vi "PH_Connection.VISA find Resources.vi"(5 "error in":errorcluster) -> (16 "VISA Information":T1(array[cluster]) {"Interface Information: Interface Type" items=["GPIB"=1, "VXI"=2, "GPIB-VXI"=3, "Serial"=4, "PXI"=5, "TCPIP"=6, "USB"=7, "FireWire"=9]}, 19 "error out":errorcluster)   [LabVIEW 2014, in "PH_Common.lvlib"]
doc: "This VI is forseen to select a string from an array of strings."
uses:
  PH_Common.lvlib
panel:
  in  "Find VISA Resources":bool
  in  "STOP":bool
  # "PCS"
  # "3.40"
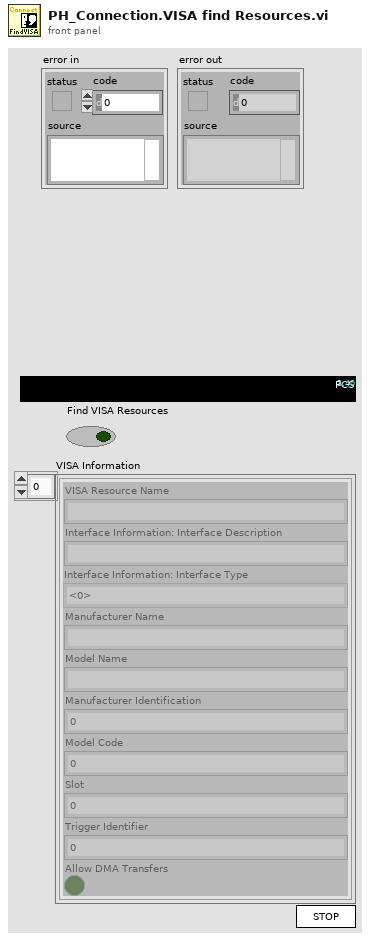
[diagram p1: front panel]
types:
  T1 = cluster{"VISA Resource Name":string, "Interface Information: Interface Description":string, "Interface Information: Interface Type":u16, "Manufacturer Name":string, "Model Name":string, "Manufacturer Identification":u16, "Model Code":u16, "Slot":i16, "Trigger Identifier":i16, "Allow DMA Transfers":bool}[]
  T2 = cluster{"VISA Resource Name":string, "Manufacturer Name":string, "Model Name":string, "Manufacturer Identification":u16, "Model Code":u16, "Slot":i16, "Trigger Identifier":i16, "Allow DMA Transfers":bool}[]
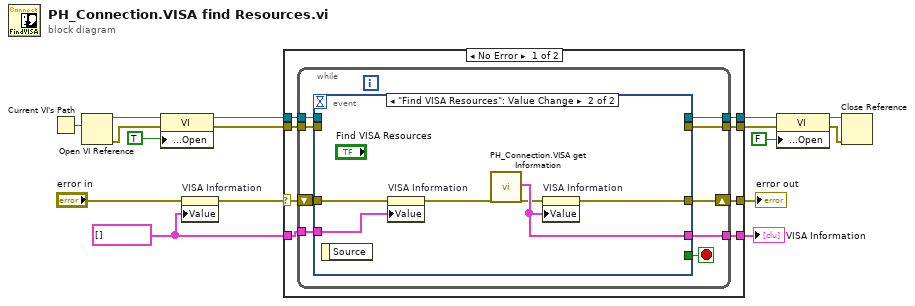
[diagram p0: block diagram]
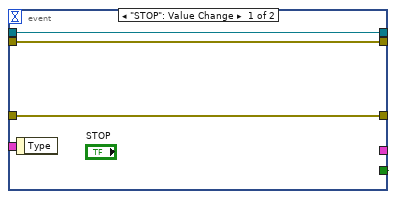
[diagram p2: hidden frame]
diagram:
  w1 = T1 [] ("VISA Information")
  n1 = Current VI's Path() -> (path=w15:path)
  n2 = Open VI Reference(vi path=w15) -> (vi reference=w14:refnum<vi>, error out=w8:errorcluster)  [unwired: 5 in]
  n3 = property class="VI"(reference=w14, error in=w8, "Front Panel Window:Open"=TRUE) -> (reference out=w12:refnum<vi>, error out=w6:errorcluster)
  n4 = property on="VISA Information" class="Arr (strict)"(error in="error in", "Value"=w1) -> (error out=w2:errorcluster)  [unwired: 1 in, 1 out]
  n5 = case shown="No Error" w2 {
    selector: w2 -> [w21 w47]
    tunnel: [w22 w47] -> w16
    tunnel: w12 -> [w24 w46]
    tunnel: [w23 w46] -> w10
    tunnel: w6 -> [w20 w45]
    tunnel: [w19 w45] -> w5
    tunnel: [w18 w44] -> w4
    tunnel: w1 -> [w17 w44]
    frame No Error {
      n6 = while {
        tunnel: w24 -> [w33]
        tunnel: [w32] -> w23
        shift-right: [w31] -> w22
        shift-left: w21 -> [w30]
        tunnel: w20 -> [w28]
        tunnel: [w27] -> w19
        tunnel: [w26] -> w18
        tunnel: w17 -> [w25]
        stop <- w29 stop-if-true
        n7 = event shown="[1] \"Find VISA Resources\": Value Change" {
          selector: _ -> [_ _]
          dyn-events: _ -> [_ _]
          timeout: _ -> [_ _]
          tunnel: [w37 _] -> w32
          tunnel: w33 -> [w37 _]
          tunnel: w30 -> [w36 w40]
          tunnel: [w36 w41] -> w31
          tunnel: [TRUE _] -> w29
          tunnel: w28 -> [w34 _]
          tunnel: [w34 _] -> w27
          tunnel: [_ w43] -> w26
          tunnel: w25 -> [_ w38]
          event "STOP": Value Change {
            n8 = event-data() -> ()  [unwired: 1 in, 1 out]
          }
          event "Find VISA Resources": Value Change {
            n9 = event-data() -> ()  [unwired: 1 in, 1 out]
            n10 = property on="VISA Information" class="Arr (strict)"(error in=w40, "Value"=w38) -> (error out=w39:errorcluster)  [unwired: 1 in, 1 out]
            n11 = call "PH_Connection.VISA get Information.vi"("error in"=w39) -> ("VISA Information"=w43:T1, "error out"=w42:errorcluster)  [unwired: 17 in]
            n12 = property on="VISA Information" class="Arr (strict)"(error in=w42, "Value"=w43) -> (error out=w41:errorcluster)  [unwired: 1 in, 1 out]
          }
        }
      }
    }
    frame Error {
      (unwired) T2 []
      (unwired) "N/A" ("String")
    }
  }
  "error out" <- w16
  "VISA Information" <- w4
  n13 = property class="VI"(reference=w10, error in=w5, "Front Panel Window:Open"=FALSE) -> (reference out=w9:refnum<vi>, error out=w7:errorcluster)
  n14 = Close Reference(reference=w9, error in (no error)=w7) -> ()  [unwired: 1 out]
